vi "valves_pumpinit.vi"(0 "COM4 in":refnum<k24>, 3 "error in":errorcluster) -> (5 "COM4 out":refnum<k24>, 6 "Commands out":T1, 7 "error out":errorcluster)   [LabVIEW 2018]
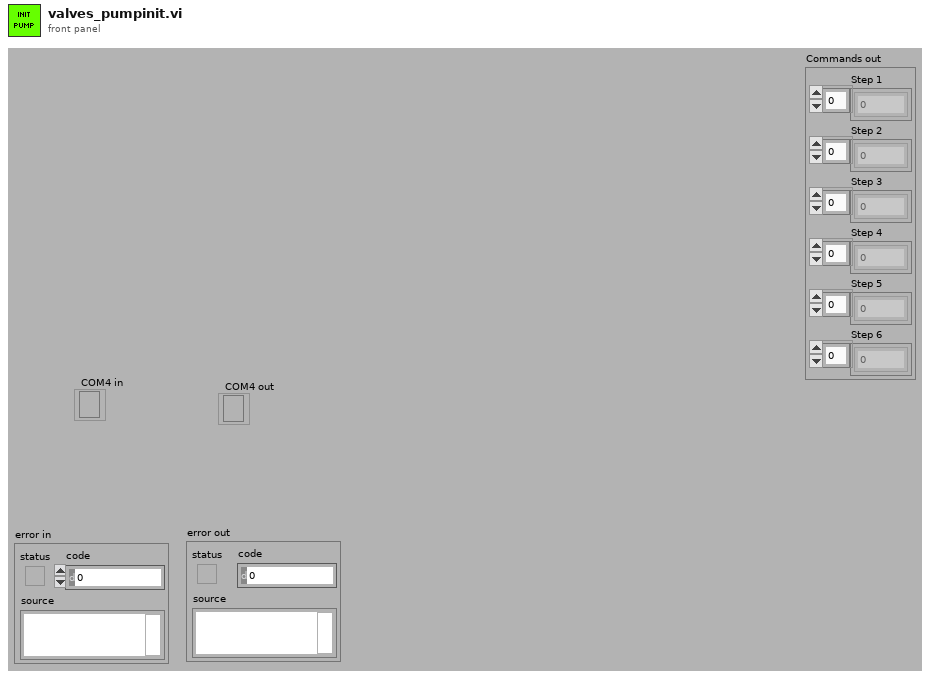
[diagram p1: front panel]
types:
  T1 = cluster{"Step 1":u8[], "Step 2":u8[], "Step 3":u8[], "Step 4":u8[], "Step 5":u8[], "Step 6":u8[]}
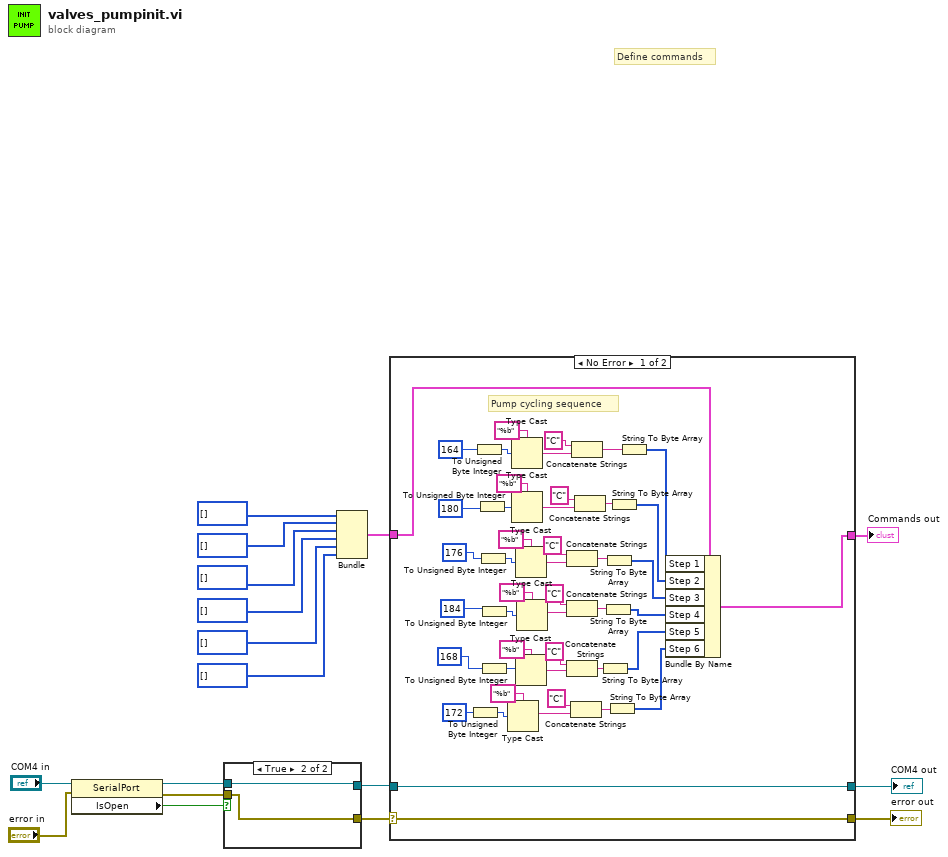
[diagram p0: block diagram]
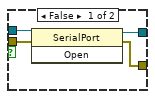
[diagram p2: hidden frame]
diagram:
  # "Define commands"
  n1 = property class="SerialPort"(reference="COM4 in", error in="error in") -> (reference out=w4:refnum<k24>, error out=w3:errorcluster, "IsOpen"=w5:bool)
  n2 = case shown="True" w5 {
    tunnel: w4 -> [w21 w22]
    tunnel: w3 -> [w20 w23]
    tunnel: [w19 w22] -> w2
    tunnel: [w18 w23] -> w1
    frame False {
      n3 = invoke class="SerialPort" method="Open"(reference=w21, error in=w20) -> (reference out=w19:refnum<k24>, error out=w18:errorcluster)  [unwired: 1 in, 1 out]
    }
    frame True {
    }
  }
  n4 = Bundle("Step 1"=u8[] [], "Step 2"=u8[] [], "Step 3"=u8[] [], "Step 4"=u8[] [], "Step 5"=u8[] [], "Step 6"=u8[] []) -> (w8:T1)  [unwired: 1 in]
  n5 = case shown="No Error" w1 {
    selector: w1 -> [w47 w71]
    tunnel: [w45 w70] -> w9
    tunnel: [w47 w71] -> w17
    tunnel: w2 -> [w46 w72]
    tunnel: [w46 w72] -> w16
    tunnel: w8 -> [w24 w70]
    frame No Error {
      # "Pump cycling sequence"
      n6 = To Unsigned Byte Integer(number=u8 172) -> (unsigned 8bit integer=w65:u8)
      n7 = To Unsigned Byte Integer(number=u8 164) -> (unsigned 8bit integer=w48:u8)
      n8 = To Unsigned Byte Integer(number=u8 180) -> (unsigned 8bit integer=w52:u8)
      n9 = To Unsigned Byte Integer(number=u8 176) -> (unsigned 8bit integer=w56:u8)
      n10 = To Unsigned Byte Integer(number=u8 184) -> (unsigned 8bit integer=w60:u8)
      n11 = To Unsigned Byte Integer(number=u8 168) -> (unsigned 8bit integer=w39:u8)
      n12 = Type Cast(type="%b", x=w65) -> (*(type *) &x=w66:string)
      n13 = Type Cast(type="%b", x=w48) -> (*(type *) &x=w49:string)
      n14 = Type Cast(type="%b", x=w52) -> (*(type *) &x=w53:string)
      n15 = Type Cast(type="%b", x=w56) -> (*(type *) &x=w57:string)
      n16 = Type Cast(type="%b", x=w39) -> (*(type *) &x=w37:string)
      n17 = Type Cast(type="%b", x=w60) -> (*(type *) &x=w61:string)
      n18 = Concatenate Strings("C", w57) -> (w32:string)
      n19 = Concatenate Strings("C", w61) -> (w30:string)
      n20 = Concatenate Strings("C", w37) -> (w28:string)
      n21 = Concatenate Strings("C", w66) -> (w26:string)
      n22 = Concatenate Strings("C", w49) -> (w36:string)
      n23 = Concatenate Strings("C", w53) -> (w34:string)
      n24 = String To Byte Array(string=w28) -> (unsigned byte array=w27:u8[])
      n25 = String To Byte Array(string=w30) -> (unsigned byte array=w29:u8[])
      n26 = String To Byte Array(string=w32) -> (unsigned byte array=w31:u8[])
      n27 = String To Byte Array(string=w26) -> (unsigned byte array=w25:u8[])
      n28 = String To Byte Array(string=w34) -> (unsigned byte array=w33:u8[])
      n29 = String To Byte Array(string=w36) -> (unsigned byte array=w35:u8[])
      n30 = Bundle By Name(cluster=w24, "Step 1"=w35, "Step 2"=w33, "Step 3"=w31, "Step 4"=w29, "Step 5"=w27, "Step 6"=w25) -> (w45:T1)
    }
    frame Error {
    }
  }
  "error out" <- w17
  "COM4 out" <- w16
  "Commands out" <- w9
